vi "Enable Auto Sequence Mode.vi"(8 "error in (no error)":errorcluster, 9 "Memory":u32(ring) items=["Not Available", "Available"], 10 "Enable Auto Sequence Mode":bool, 11 "VISA resource name":refnum<visa-resource-name>="TCPIP0::192.168.0.200::50505::SOCKET") -> (0 "error out":errorcluster, 3 "VISA resource name out":refnum<visa-resource-name>="TCPIP0::192.168.0.200::50505::SOCKET")   [LabVIEW 2022 SP3, in "MagnaDC.lvlib"]
uses:
  MagnaDC.lvlib
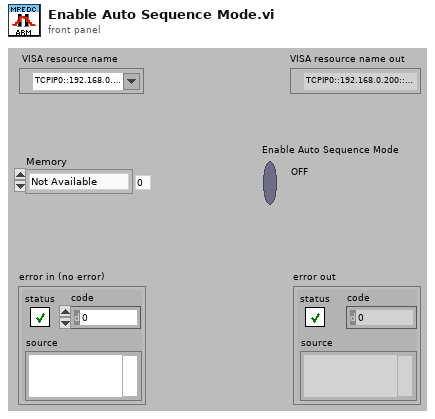
[diagram p1: front panel]
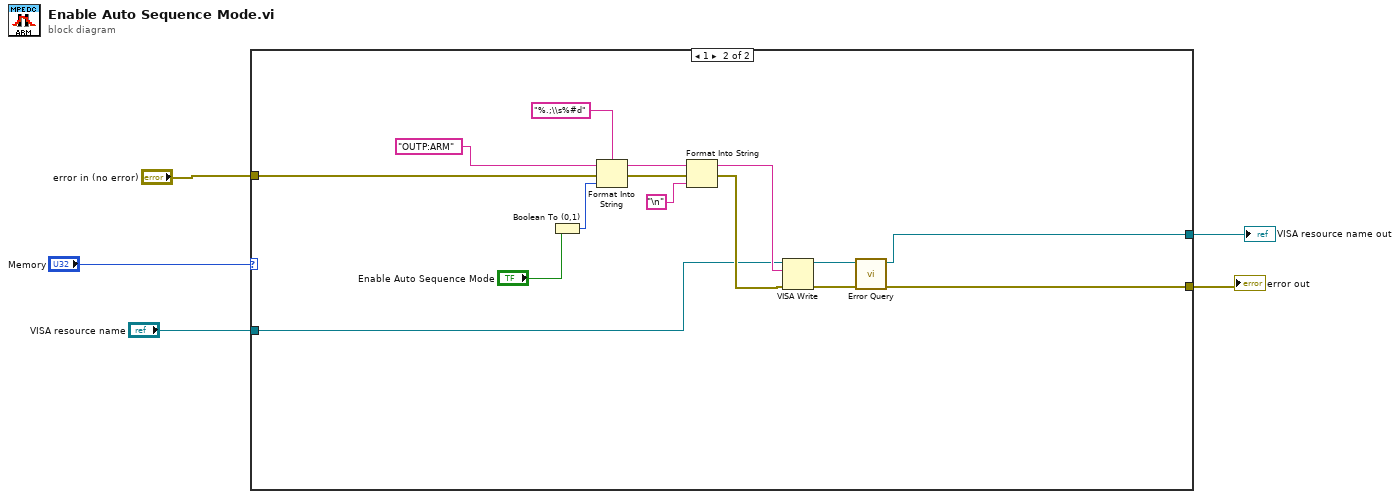
[diagram p0: block diagram]
diagram:
  n1 = case shown="1" "Memory" {
    tunnel: "VISA resource name" -> [w6 w11]
    tunnel: "error in (no error)" -> [w7 w10]
    tunnel: [w6 w9] -> w2
    tunnel: [w7 w8] -> w1
    frame 0, Default {
    }
    frame 1 {
      n2 = Boolean To (0,1)(Boolean="Enable Auto Sequence Mode") -> (0, 1=w22:i16)
      n3 = Format Into String(format string="%.;\\s%#d", initial string="OUTP:ARM", error in=w10, w22) -> (resulting string=w21:string, error out=w20:errorcluster)
      n4 = Format Into String(initial string=w21, error in=w20, "\n") -> (resulting string=w18:string, error out=w19:errorcluster)  [unwired: 1 in]
      n5 = VISA Write(VISA resource name=w11, write buffer=w18, error in (no error)=w19) -> (VISA resource name out=w15:refnum<visa-resource-name>, error out=w16:errorcluster)  [unwired: 1 out]
      n6 = call "Error Query.vi"("error in (no error)"=w16, "VISA resource name"=w15) -> ("error out"=w8:errorcluster, "VISA resource name out"=w9:refnum<visa-resource-name>)  [unwired: 6 in, 2 out]
    }
  }
  "VISA resource name out" <- w2
  "error out" <- w1
